vi "Measurement Logic.vi"() -> ()   [LabVIEW 2020, in "NIFgenStandardFunction.lvlib"]
uses:
  NIFgenStandardFunction.lvlib
  Measurement Configuration.ctl
  Waveform.ctl
  Measurement Results.ctl
  <vilib>/MeasurementLink/MeasurementLink Measurement Server/Classes/MeasurementContext/MeasurementContext.lvclass
  <vilib>/MeasurementLink/MeasurementLink Measurement Server/Classes/MeasurementContext/Reserve Sessions - 1Pin.vi
  <vilib>/MeasurementLink/MeasurementLink niFGEN/Create Sessions - 1Sess.vi
  <vilib>/MeasurementLink/MeasurementLink niFGEN/MeasurementLink niFGEN.lvlib
  <vilib>/MeasurementLink/MeasurementLink Session Management/Session Reservation/Session Reservation.lvclass
panel:
  out "Measurement Context out":refnum<class "MeasurementContext.lvclass">
  in  "Measurement Context":refnum<class "MeasurementContext.lvclass">
  out "Measurement Results":T1={"actual_duration"=1.0}
  in  "Measurement Configuration":T2={"pin_name"="", "waveform"=enum."Noise", "frequency"=6.0, "amplitude"=6.0, "duration"=6.0}
  out "error out":errorcluster
  in  "error in":errorcluster
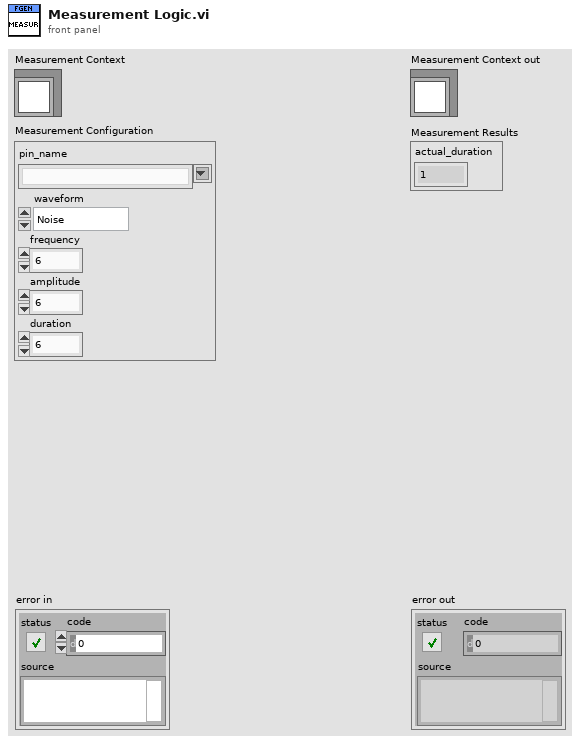
[diagram p1: front panel]
types:
  T1 = typedef "NIFgenStandardFunction.lvlib/Measurement Results.ctl" = cluster{"actual_duration":dbl}
  T2 = typedef "NIFgenStandardFunction.lvlib/Measurement Configuration.ctl" = cluster{"pin_name":string, "waveform":T3, "frequency":dbl, "amplitude":dbl, "duration":dbl}
  T3 = typedef "NIFgenStandardFunction.lvlib/Waveform.ctl" = enum16{"Sine", "Square", "Triangle", "Ramp Up", "Ramp Down", "DC", "Noise", "User"}
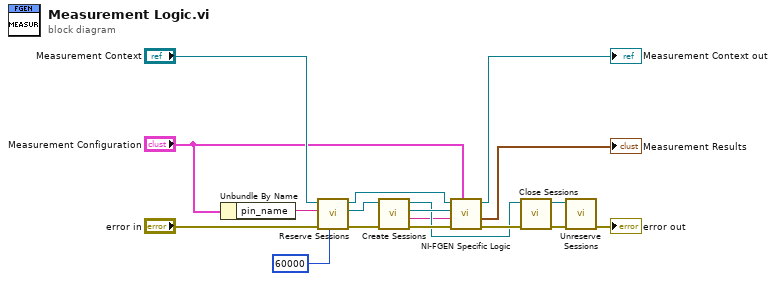
[diagram p0: block diagram]
diagram:
  n1 = Unbundle By Name("Measurement Configuration") -> ("pin_name"=w17:string)
  n2 = call-poly <vilib>:"Reserve Sessions.vi"("timeout (ms)"=60000, "error in"="error in", "pin or relay name"=w17, "measurement context in"="Measurement Context") -> ("error out"=w10:errorcluster, "session reservation out"=w9:refnum<class "Session Reservation.lvclass">, "measurement context out"=w12:refnum<class "MeasurementContext.lvclass">)  [unwired: 5 in]
  n3 = call-poly <vilib>:"Create Sessions.vi"("error in"=w10, "session reservation in"=w9) -> ("error out"=w15:errorcluster, "channel list"=w2:string, "session"=w13:refnum<k15>, "session reservation out"=w6:refnum<class "Session Reservation.lvclass">)  [unwired: 6 in]
  n4 = call "NI-FGEN Specific Logic.vi"("measurement configuration"="Measurement Configuration", "error in"=w15, "channel list"=w2, "session"=w13, "measurement context"=w12) -> ("error out"=w7:errorcluster, "measurement results"=→"Measurement Results":T1, "measurement context out"=→"Measurement Context out":refnum<class "MeasurementContext.lvclass">)  [unwired: 3 in, 1 out]
  n5 = call <vilib>:"Close Sessions.vi"("error in"=w7, "session reservation in"=w6) -> ("error out"=w5:errorcluster, "session reservation out"=w4:refnum<class "Session Reservation.lvclass">)  [unwired: 8 in]
  n6 = call <vilib>:"Unreserve Sessions.vi"("error in"=w5, "session reservation in"=w4) -> ("error out"=→"error out":errorcluster)  [unwired: 9 in]
